vi "GetTerms3.vi"(0 "XRef":T10, 1 "State In":T9={"Output Type"=variant(dbl 0.0), "Typedef Name"="", "Input Type"=variant, "Constant Types"=[], "Error"={"status"=FALSE, "code"=0, "source"=""}, "Typedef Path"=path "", "Names"=[], "Event Cluster Name"=""}) -> (14 "Terms":T1)   [LabVIEW 2015, in "Create-Signals.xnode"]
doc: "This ability VI is used to describe your terminals to LabVIEW. Terms is an array of clusters describing the XNode's terminals.\n ID: A unique string identifying the terminal.\n Name: The name of the terminal visible to the user. Remember to localize it.\n Type: The data type of the terminal (as a Variant). The data put in the variant will be used as the default for the input terminal if it's left unwired.\n Bounds: A rectangle defining the bounds of the terminal relative to the bounds of the XNode. The bounds must be within the bounds of the XNode, and for whiskers to draw properly, they must be flush with at least one side of the XNode.\n Input?: Indicates whether or not this terminals is an input.\n Required?: Indicates whether the user must wire this terminal for the XNode to not be broken. Ignored on outputs.\n Recommended?: Indicates whether the terminal is recommended.\n Hidden?: Indicates whether the terminal is hidden. When a terminal is hidden, it cannot be wired to via user interaction or scripting. However, if it is already wired to when the hidden flag is changed to true, it will remain wired.\n Adaptive?: Indicates that the term should change to match the type of its source if it is wired.\n Direction?: Indicates what direction the wire stub should point. Choose auto to let LV decide based on the terms bounds being on the nodes edge.\n \n The IDs are used by LabVIEW to keep track of your terminals. When you respecify your terminals, LabVIEW can tell whther terminals are new, deleted, or moved by the unique IDs. The order is irrelevant. If you move a terminal, then any wire connected to it will move with it.\n \n If you want to update your terminals, you should return the UpdateTerms reply in one of your ability VIs.\n\nDefault behavior: None.\n\nThis ability does not provide UI and OS messages are not handled."
uses:
  Create-Signals.xnode
  <vilib>/XNodeSupport/XNodeXNodeRef.ctl
  State.ctl
  <vilib>/XNodeSupport/XNodeTerm3Array.ctl
  <vilib>/XNodeSupport/XNodeTerm3.ctl
  <vilib>/XNodeSupport/XNodeString.ctl
  <vilib>/XNodeSupport/XNodeVariant.ctl
  <vilib>/XNodeSupport/XNodeRect32.ctl
  <vilib>/XNodeSupport/XNodeInt.ctl
  <vilib>/XNodeSupport/XNodeBool.ctl
  <vilib>/XNodeSupport/XNodeTermDirection.ctl
  <vilib>/XNodeSupport/NI_XNodeSupport.lvlib
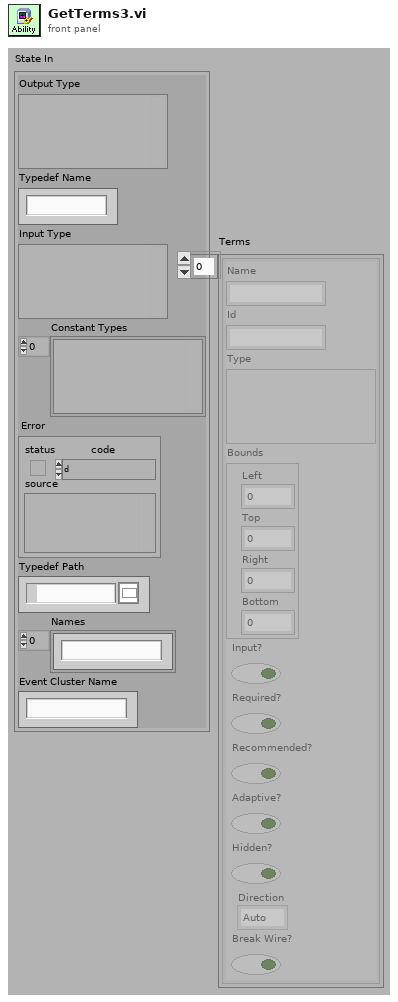
[diagram p1: front panel]
types:
  T1 = typedef "NI_XNodeSupport.lvlib/XNodeTerm3Array.ctl" = T2[]
  T2 = typedef "NI_XNodeSupport.lvlib/XNodeTerm3.ctl" = cluster{"Name":T3, "Id":T3, "Type":T4, "Bounds":T5, "Input?":T7, "Required?":T7, "Recommended?":T7, "Adaptive?":T7, "Hidden?":T7, "Direction":T8, "Break Wire?":T7}
  T3 = typedef "NI_XNodeSupport.lvlib/XNodeString.ctl" = string
  T4 = typedef "NI_XNodeSupport.lvlib/XNodeVariant.ctl" = variant
  T5 = typedef "NI_XNodeSupport.lvlib/XNodeRect32.ctl" = cluster{"Left":T6, "Top":T6, "Right":T6, "Bottom":T6}
  T6 = typedef "NI_XNodeSupport.lvlib/XNodeInt.ctl" = i32
  T7 = typedef "NI_XNodeSupport.lvlib/XNodeBool.ctl" = bool
  T8 = typedef "NI_XNodeSupport.lvlib/XNodeTermDirection.ctl" = enum32{"Auto", "Up", "Down", "Left", "Right", "Center"}
  T9 = typedef "Create-Signals.xnode/State.ctl" = cluster{"Output Type":variant, "Typedef Name":string, "Input Type":variant, "Constant Types":variant[], "Error":errorcluster, "Typedef Path":path, "Names":string[], "Event Cluster Name":string}
  T10 = typedef "NI_XNodeSupport.lvlib/XNodeXNodeRef.ctl" = refnum<vi>
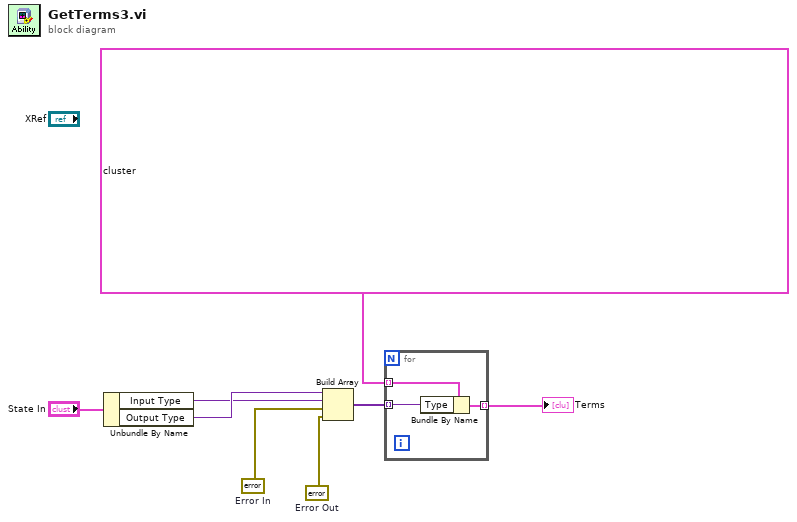
[diagram p0: block diagram]
diagram:
  w6 = errorcluster {"status"=FALSE, "code"=0, "source"=""}  # Error Out
  w7 = errorcluster {"status"=FALSE, "code"=0, "source"=""}  # Error In
  n1 = Unbundle By Name("State In") -> ("Input Type"=w3:variant, "Output Type"=w4:variant)
  n2 = Build Array(w4, w3, w7, w6) -> (w8:variant[])
  n3 = for {
    tunnel: T2[] [{"Name"="Signals", "Id"="out", "Type"=variant, "Bounds"={"Left"=24, "Top"=0, "Right"=32, "Bottom"=8}, "Input?"=FALSE, "Required?"=FALSE, "Recommended?"=TRUE, "Adaptive?"=TRUE, "Hidden?"=FALSE, "Direction"=enum."Auto", "Break Wire?"=FALSE}, {"Name"="Values", "Id"="in", "Type"=variant, "Bounds"={"Left"=0, "Top"=0, "Right"=8, "Bottom"=8}, "Input?"=TRUE, "Required?"=TRUE, "Recommended?"=TRUE, "Adaptive?"=FALSE, "Hidden?"=FALSE, "Direction"=enum."Auto", "Break Wire?"=FALSE}, {"Name"="Error In", "Id"="ein", "Type"=variant, "Bounds"={"Left"=0, "Top"=24, "Right"=8, "Bottom"=32}, "Input?"=TRUE, "Required?"=FALSE, "Recommended?"=TRUE, "Adaptive?"=FALSE, "Hidden?"=FALSE, "Direction"=enum."Auto", "Break Wire?"=FALSE}, {"Name"="Error Out", "Id"="eout", "Type"=variant, "Bounds"={"Left"=24, "Top"=24, "Right"=32, "Bottom"=32}, "Input?"=FALSE, "Required?"=FALSE, "Recommended?"=TRUE, "Adaptive?"=FALSE, "Hidden?"=FALSE, "Direction"=enum."Auto", "Break Wire?"=FALSE}] -> [w11] mode=indexing
    tunnel: w8 -> [w9] mode=indexing
    tunnel: [w10] -> w1 mode=indexing
    n4 = Bundle By Name(cluster=w11, "Type"=w9) -> (w10:T2)
  }
  "Terms" <- w1
